vi "Aplicatie virtuala.vi"() -> ()   [LabVIEW 2022 SP3]
panel:
  in  "Valva (B)":bool
  out "Putere electrica arbore":dbl format="%.3f"
  in  "Valva (A)":bool=TRUE
  out "Temperatura":dbl format="%.2f"
  out "Senzor 2":bool
  out "Senzor 1":bool
  out "Deschidere":dbl=4.710000000000006 min=0.0 max=10.0 step=0.01 format="%.2f"
  in  "Debit volumetric 2":dbl=25.39 min=0.0 max=50.0 step=0.01 format="%.2f"
  out "M 3":bool
  out "M 2":bool
  out "Timp curgere":dbl=4.710000000000006 min=0.0 max=10.0 step=0.01 format="%.2f"
  out "Viteza curgere":dbl=4.710000000000006 min=0.0 max=10.0 step=0.01 format="%.2f"
  out "M":bool
  in  "Motor":bool
  in  "?":bool
  out "Energie electrica consumata":dbl format="%.3f"
  out "Putere electrica absorbita":dbl format="%.3f"
  out "?":dbl(slide) scale=0.0..1200.0
  out "?":bool
  out "?":bool
  in  "Orificiu":bool=TRUE
  in  "?":bool
  out "?":dbl(slide) scale=0.0..1200.0 scale format="%.2f"
  out "Cantitate evacuata":dbl
  out "Debit volumetric":dbl=4.710000000000006 min=0.0 max=10.0 step=0.01 format="%.2f"
  # "Rezervor principal\n1000 l"
  # "BALAN COSMIN-STEFAN"
  # "MONITORIZARE SI CONTROL \nPROCES INDUSTRIAL\n(SENSORLESS)"
  # "0 l/s - 50 l/s"
  # "l"
  # "100%"
  # "80%"
  # "l/s"
  # "%"
  # "40%"
  # "l/s"
  # "l"
  # "m/s"
  # "1 m"
  # "Rezervor secundar\n1000 l"
  # "s"
  # "l"
  # "100%"
  # "kW"
  # "kW"
  # "80%"
  # "*C"
  # "kWh"
  # "40%"
  # "0 l/s sau 50 l/s"
  # "BALAN COSMIN-STEFAN"
  # "MONITORIZARE SI PROTECTIE \nTEMPERATURA\n(SENSORLESS)"
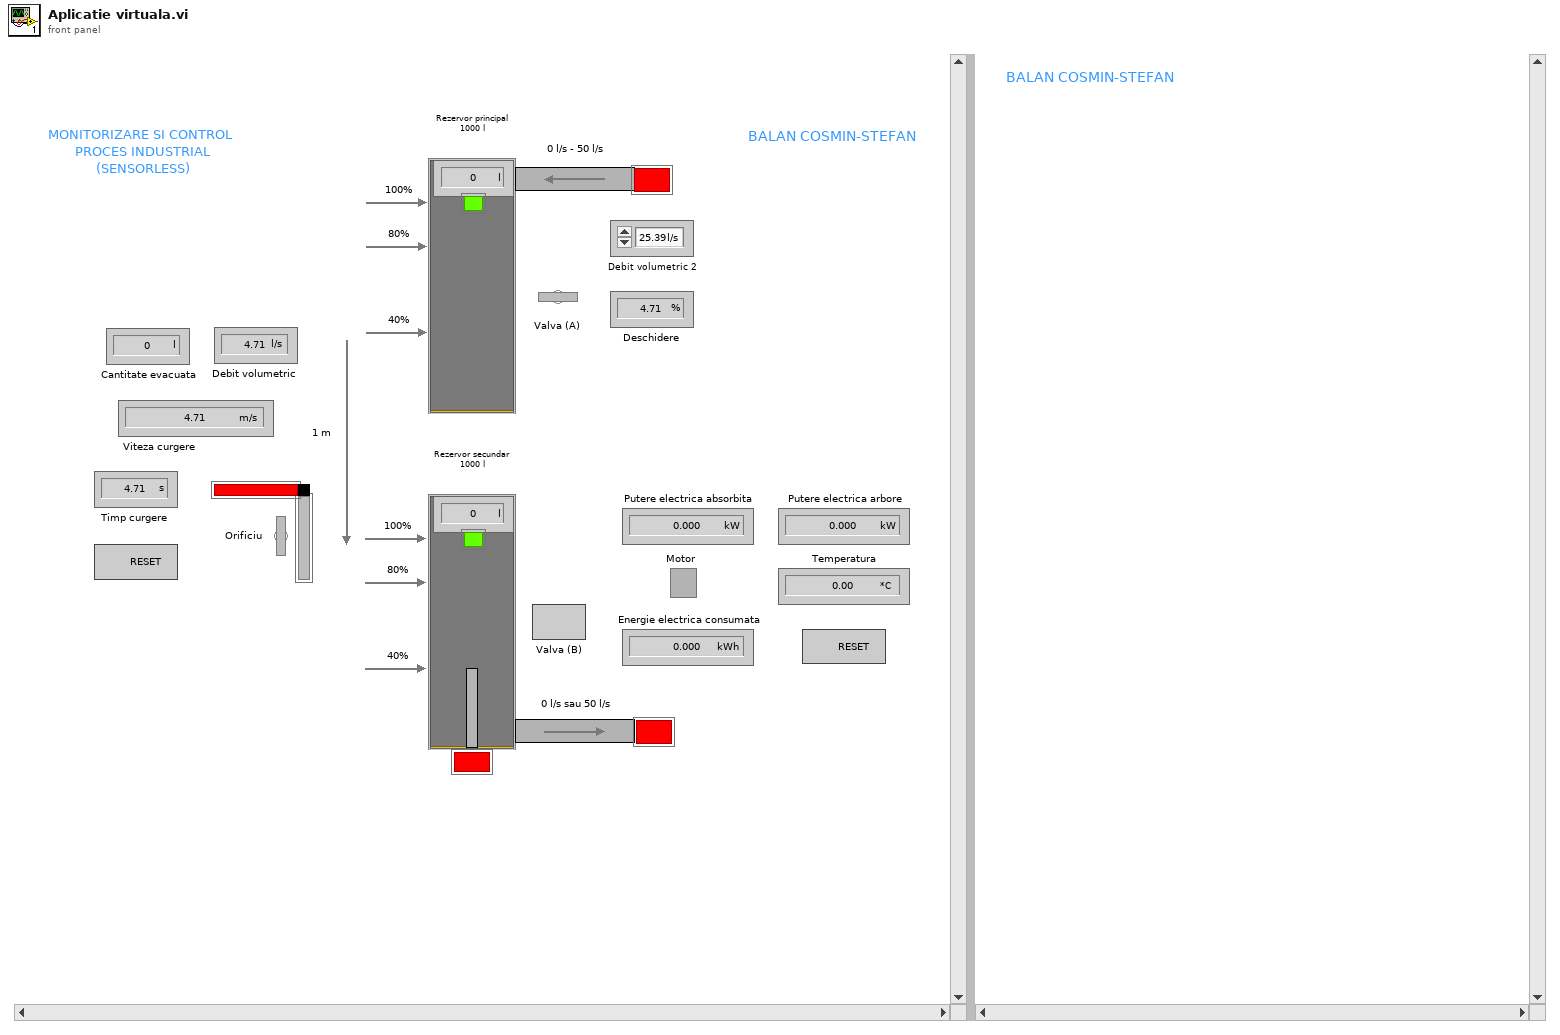
[diagram p1: front panel]
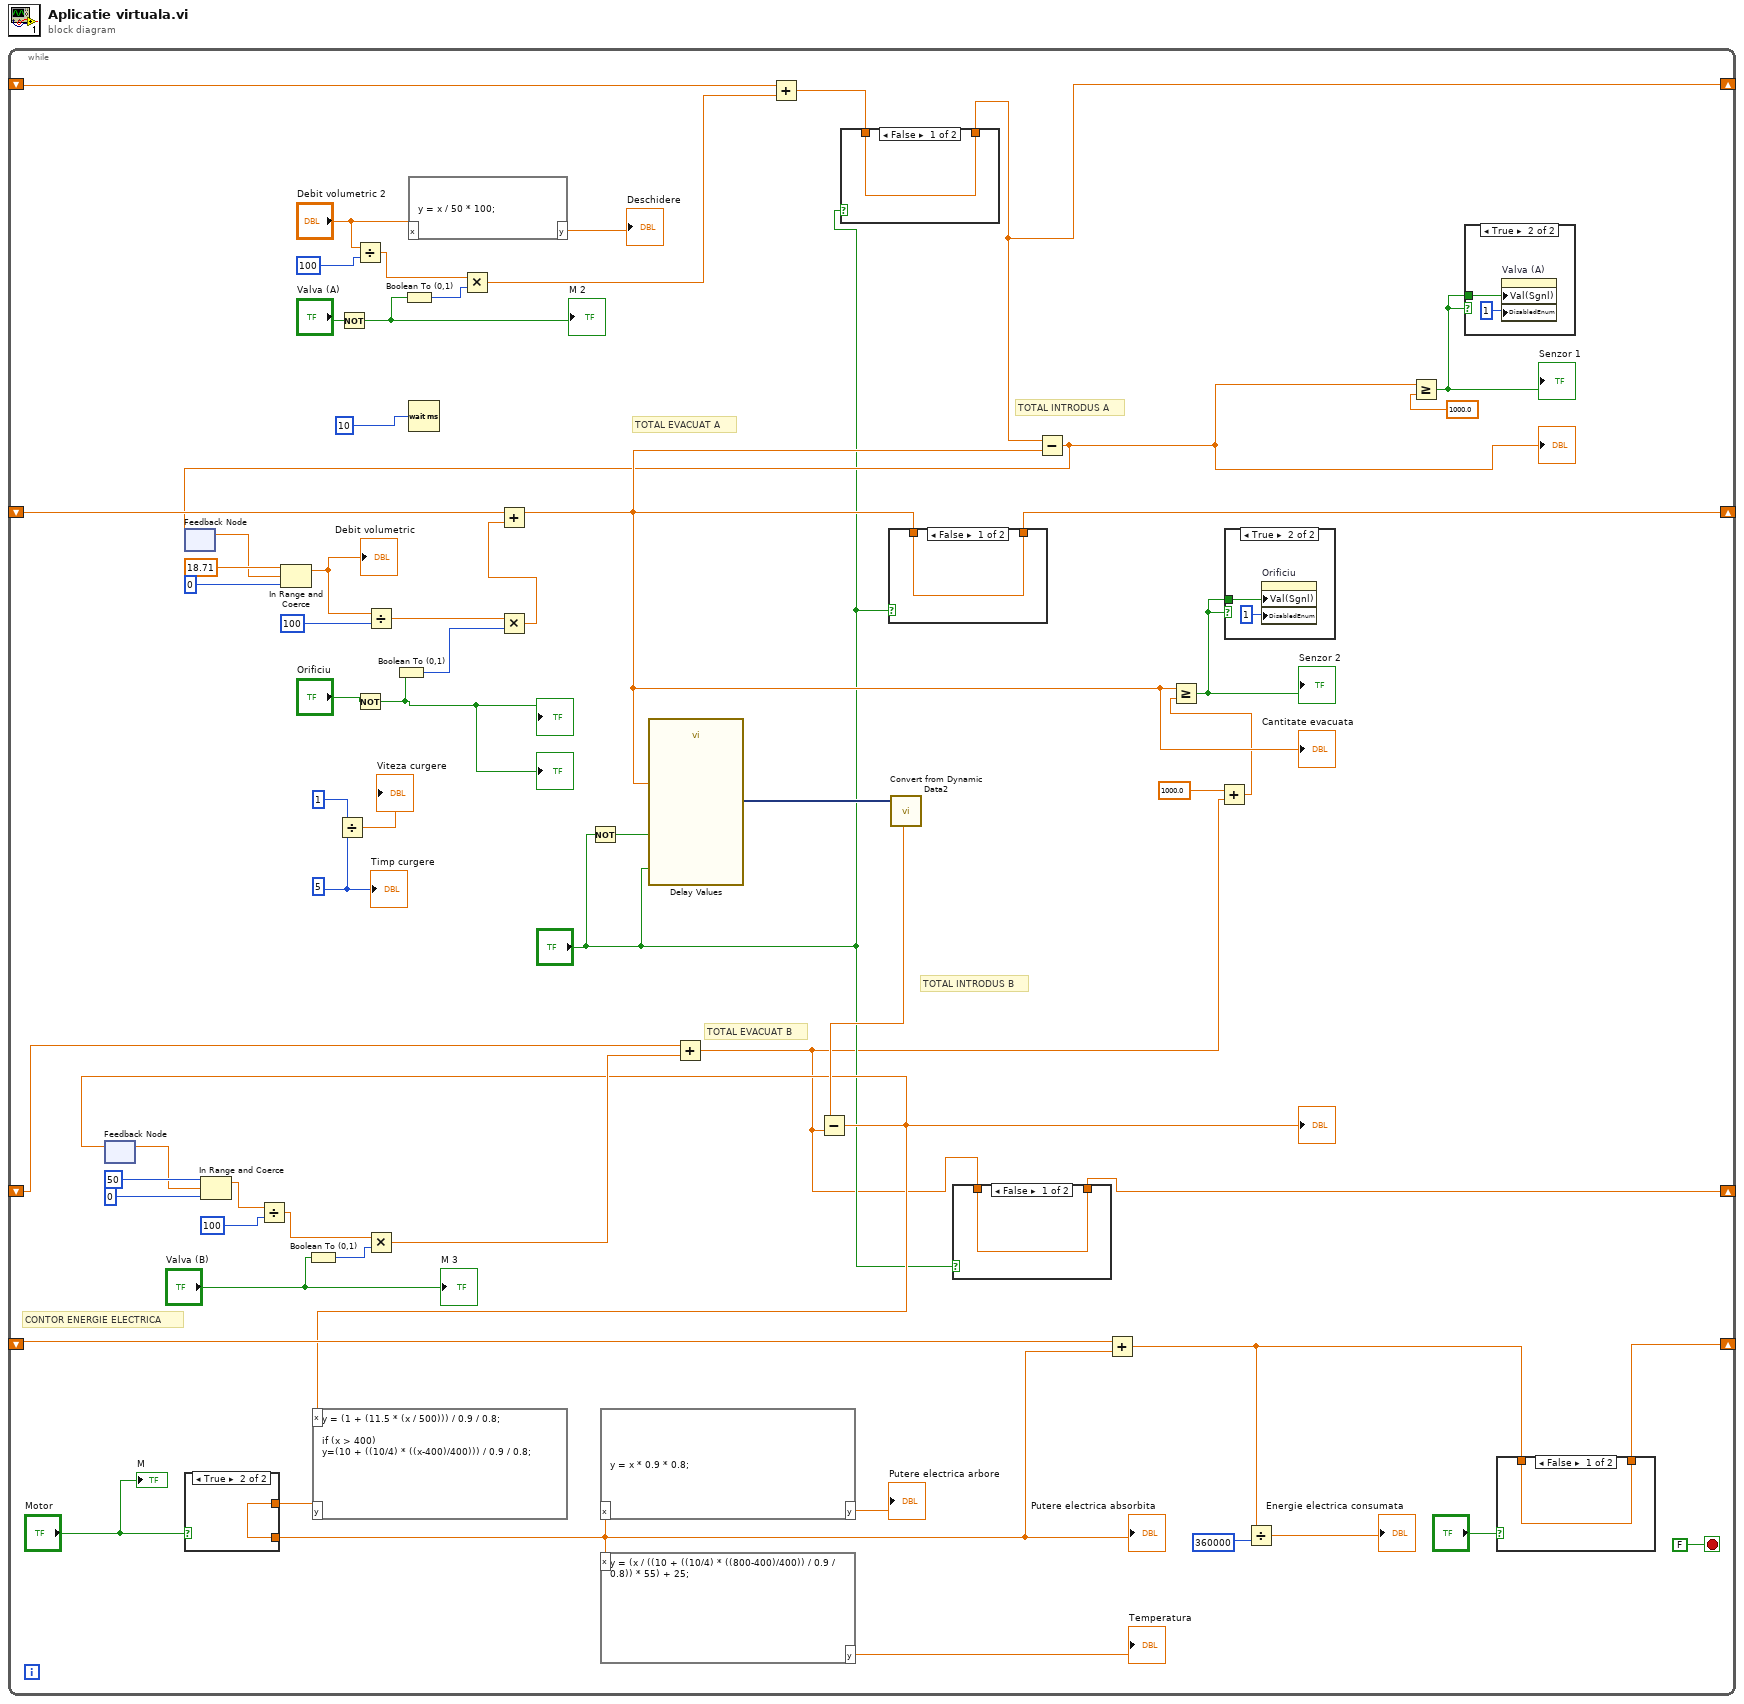
[diagram p0: block diagram]
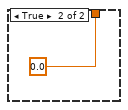
[diagram p2: hidden frame]
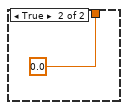
[diagram p3: hidden frame]
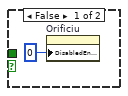
[diagram p4: hidden frame]
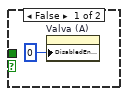
[diagram p5: hidden frame]
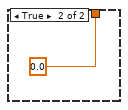
[diagram p6: hidden frame]
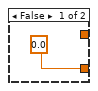
[diagram p7: hidden frame]
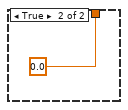
[diagram p8: hidden frame]
diagram:
  n1 = while {
    shift-right: [w61] -> _
    shift-left: _ -> [w62]
    shift-right: [w49] -> _
    shift-left: _ -> [w55]
    shift-right: [w26] -> _
    shift-left: _ -> [w37]
    shift-right: [w5] -> _
    shift-left: _ -> [w12]
    stop <- FALSE stop-if-true
    w45 = 5
    # "TOTAL EVACUAT B"
    # "TOTAL INTRODUS B"
    # "CONTOR ENERGIE ELECTRICA"
    # "TOTAL EVACUAT A"
    # "TOTAL INTRODUS A"
    n2 = feedback #1() -> (w9:dbl)  [unwired: 1 in]
    n3 = feedback #2() -> (w22:dbl)  [unwired: 1 in]
    n4 = In Range and Coerce(upper limit=50, x=w9, lower limit=0) -> (coerced(x)=w8:dbl)  [unwired: 1 out]
    n5 = Divide(x=w8, y=100) -> (x/y=w14:dbl)
    n6 = In Range and Coerce(upper limit=18.71, x=w22, lower limit=0) -> (coerced(x)=w23:dbl)  [unwired: 1 out]
    "Debit volumetric" <- w23
    n7 = Boolean To (0,1)(Boolean="Valva (B)") -> (0, 1=w16:i16)
    n8 = Divide(x=1, y=w45) -> (x/y=→"Viteza curgere":dbl)
    n9 = Not(x="Valva (A)") -> (.not. x?=w36:bool)
    "M 2" <- w36
    n10 = Divide(x="Debit volumetric 2", y=100) -> (x/y=w33:dbl)
    n11 = Not(x="Orificiu") -> (.not. x?=w51:bool)
    "?" <- w51
    "?" <- w51
    n12 = Divide(x=w23, y=100) -> (x/y=w56:dbl)
    n13 = Multiply(x=w14, y=w16) -> (x*y=w15:dbl)
    n14 = Boolean To (0,1)(Boolean=w51) -> (0, 1=w59:i16)
    n15 = Boolean To (0,1)(Boolean=w36) -> (0, 1=w35:i16)
    n16 = formula code="y = x / 50 * 100;"("x"="Debit volumetric 2") -> ("y"=→"Deschidere":dbl)
    n17 = Wait (ms)(milliseconds to wait=10) -> ()  [unwired: 1 out]
    n18 = Multiply(x=w33, y=w35) -> (x*y=w34:dbl)
    n19 = Multiply(x=w56, y=w59) -> (x*y=w30:dbl)
    n20 = Add(x=w62, y=w30) -> (x+y=w29:dbl)
    "Cantitate evacuata" <- w29
    n21 = Not(x="?") -> (.not. x?=w58:bool)
    n22 = call "Delay Values"("Reset"="?", "Enable"=w58, "Signals"=w29) -> ("Delayed Signals"=w39:dynamicdata)  [unwired: 7 in, 1 out]
    n23 = Add(x=w12, y=w15) -> (x+y=w2:dbl)
    n24 = Add(x=w37, y=w34) -> (x+y=w27:dbl)
    n25 = case shown="False" "?" {
      tunnel: [w66 0.0] -> w26
      tunnel: w27 -> [w66 _]
      frame False {
      }
      frame True {
      }
    }
    n26 = case shown="False" "?" {
      tunnel: [w78 0.0] -> w61
      tunnel: w29 -> [w78 _]
      frame False {
      }
      frame True {
      }
    }
    n27 = call "Convert from Dynamic Data2"("Dynamic Data Type"=w39) -> ("Scalar"=w17:dbl)  [unwired: 3 in]
    n28 = Subtract(x=w17, y=w2) -> (x-y=w7:dbl)
    "?" <- w7
    n29 = feedback-in #1(w7) -> ()
    n30 = formula code="y = (1 + (11.5 * (x / 500))) / 0.9 / 0.8;\n\nif (x > 400)\ny=(10 + ((10/4) * ((x-400)/400))) / 0.9 / 0.8;"("x"=w7) -> ("y"=w50:dbl)
    n31 = case shown="True" "Motor" {
      tunnel: [0.0 w77] -> w19
      tunnel: w50 -> [_ w77]
      frame False {
      }
      frame True {
      }
    }
    "Putere electrica absorbita" <- w19
    n32 = formula code="y = x * 0.9 * 0.8;"("x"=w19) -> ("y"=→"Putere electrica arbore":dbl)
    n33 = formula code="y = (x / ((10 + ((10/4) * ((800-400)/400)) / 0.9 / 0.8)) * 55) + 25;"("x"=w19) -> ("y"=→"Temperatura":dbl)
    n34 = case shown="False" "?" {
      tunnel: [w64 0.0] -> w5
      tunnel: w2 -> [w64 _]
      frame False {
      }
      frame True {
      }
    }
    n35 = Subtract(x=w26, y=w29) -> (x-y=w18:dbl)
    "?" <- w18
    n36 = feedback-in #2(w18) -> ()
    n37 = Add(x=w55, y=w19) -> (x+y=w21:dbl)
    n38 = Add(x=1000.0, y=w2) -> (x+y=w1:dbl)
    n39 = Greater Or Equal?(x=w29, y=w1) -> (x >= y?=w40:bool)
    "Senzor 2" <- w40
    n40 = case shown="True" w40 {
      tunnel: w40 -> [_ w70]
      frame False {
        n41 = property on="Orificiu" class="Bool (strict)"("DisabledEnum"=0) -> ()  [unwired: 2 in, 2 out]
      }
      frame True {
        n42 = property on="Orificiu" class="Bool (strict)"("Val(Sgnl)"=w70, "DisabledEnum"=1) -> ()  [unwired: 2 in, 2 out]
      }
    }
    n43 = Divide(x=w21, y=360000) -> (x/y=→"Energie electrica consumata":dbl)
    n44 = Greater Or Equal?(x=w18, y=1000.0) -> (x >= y?=w41:bool)
    "Senzor 1" <- w41
    n45 = case shown="True" w41 {
      tunnel: w41 -> [_ w73]
      frame False {
        n46 = property on="Valva (A)" class="Bool (strict)"("DisabledEnum"=0) -> ()  [unwired: 2 in, 2 out]
      }
      frame True {
        n47 = property on="Valva (A)" class="Bool (strict)"("Val(Sgnl)"=w73, "DisabledEnum"=1) -> ()  [unwired: 2 in, 2 out]
      }
    }
    n48 = case shown="False" "?" {
      tunnel: [w74 0.0] -> w49
      tunnel: w21 -> [w74 _]
      frame False {
      }
      frame True {
      }
    }
    "M" <- "Motor"
    "Timp curgere" <- w45
    "M 3" <- "Valva (B)"
  }
